vi "Apply.vi"(8 "error in (no error)":errorcluster, 11 "Generate DC CFG in":refnum<class "Generate DC CFG.lvclass">) -> (0 "error out":errorcluster, 3 "Generate DC CFG out":refnum<class "Generate DC CFG.lvclass">)   [LabVIEW 2023, in "FGen Simulated CFGs.lvlib" / "Generate DC CFG.lvclass"]
uses:
  Generate DC CFG.lvclass
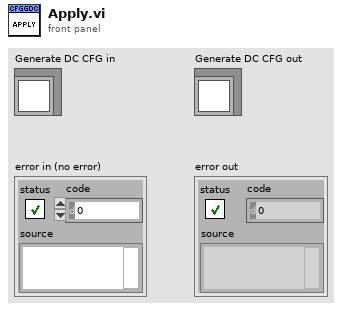
[diagram p1: front panel]
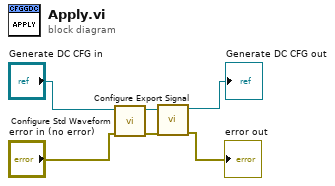
[diagram p0: block diagram]
diagram:
  n1 = call-dynamic "Configure Std Waveform.vi"("error in (no error)"="error in (no error)", "FGen PXI Base CFG in"="Generate DC CFG in") -> ("error out"=w5:errorcluster, "FGen PXI Base CFG out"=w6:refnum<class "Generate DC CFG.lvclass">)  [unwired: 8 in]
  n2 = call "Configure Export Signal.vi"("error in (no error)"=w5, "FGen PXI Base CFG in"=w6) -> ("error out"=→"error out":errorcluster, "FGen PXI Base CFG out"=→"Generate DC CFG out":refnum<class "Generate DC CFG.lvclass">)  [unwired: 8 in]
